vi "EnFlo_Seeder_Control.vi"(0 "Current Time (s)":dbl) -> ()   [LabVIEW 2021]
panel:
  in  "Minium Seeder power setting (Pmin)":dbl=27.0
  in  "Minimum Transducer Setting (Tmin)":dbl=6.0
  in  "Fluid Flowrate Factor":dbl=1.2 min=0.2 max=4.0 step=0.1 format="%.1g"
  in  "Sugar Strength":dbl=0.23
  out "Set All Outputs to Zero":bool
  in  "Performing hand clean":bool
  out "Run Transducer":bool
  out "Sugar Pump":bool
  out "Low Flow":bool
  out "High Flow":bool
  out "Time Since Last Flush (min)":dbl
  out "Running Flush time":dbl
  out "Transducer setting":dbl
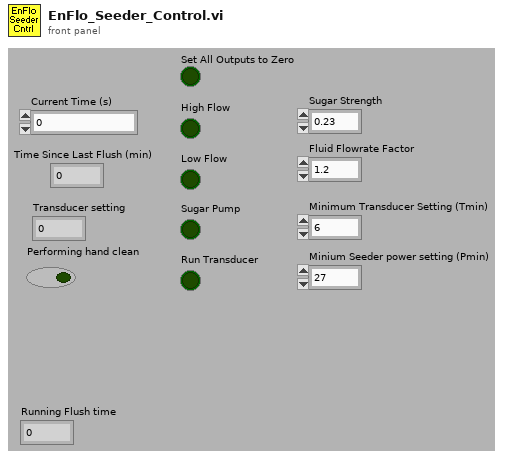
[diagram p1: front panel]
types:
  T1 = typedef "LVDateTimeRec.ctl" = cluster{"fractional second":dbl, "second":i32, "minute":i32, "hour":i32, "day of month":i32, "month":i32, "year":i32, "day of week":i32, "day of year":i32, "DST":i32}
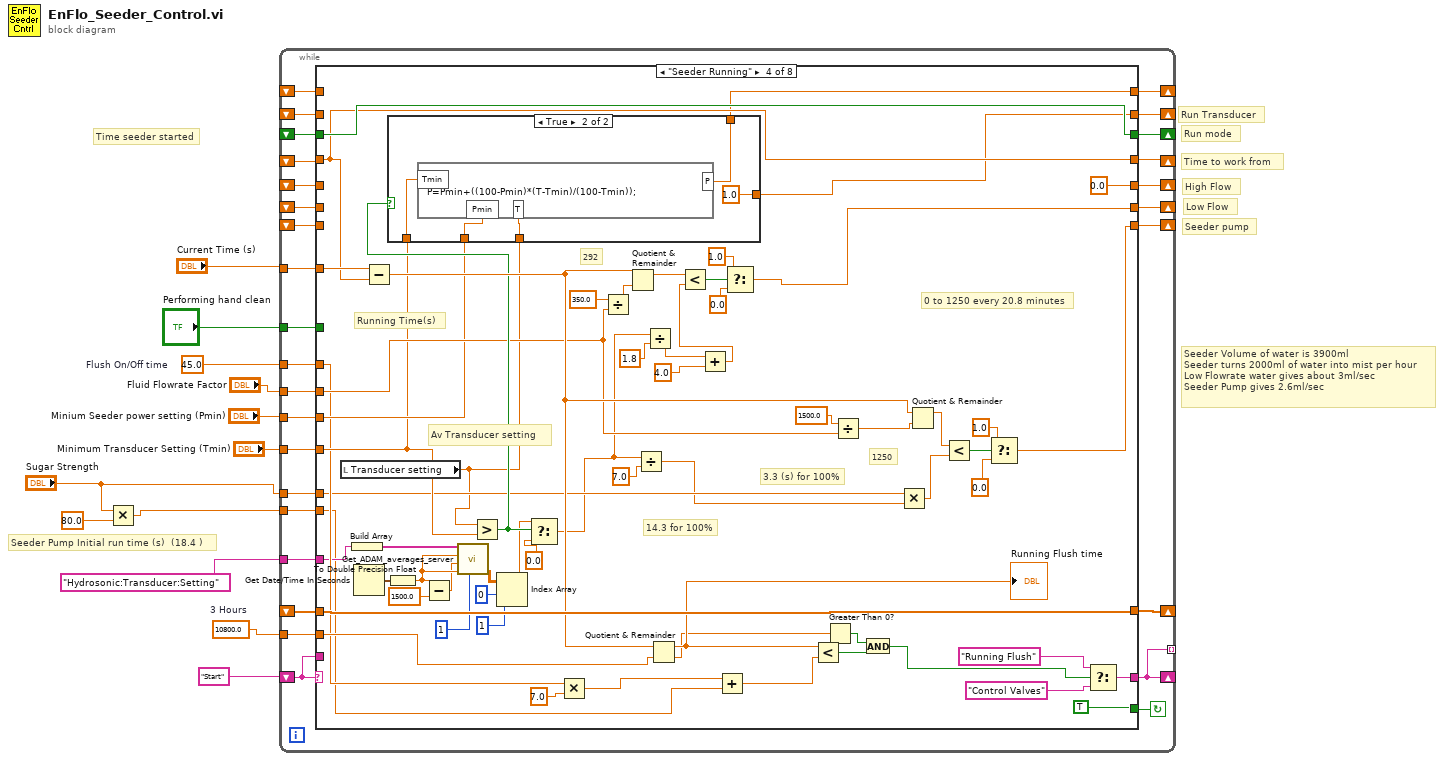
[diagram p0: block diagram]
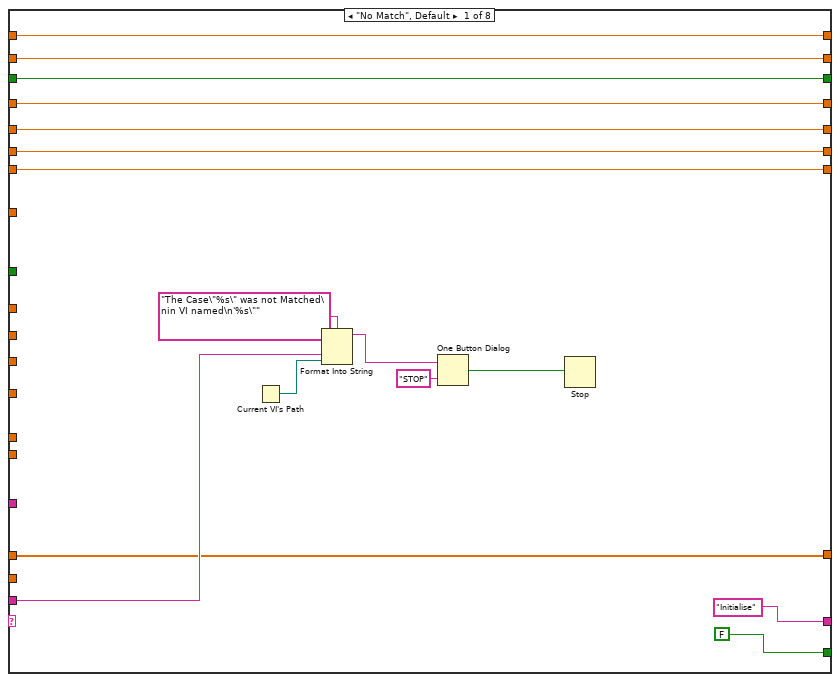
[diagram p2: hidden frame]
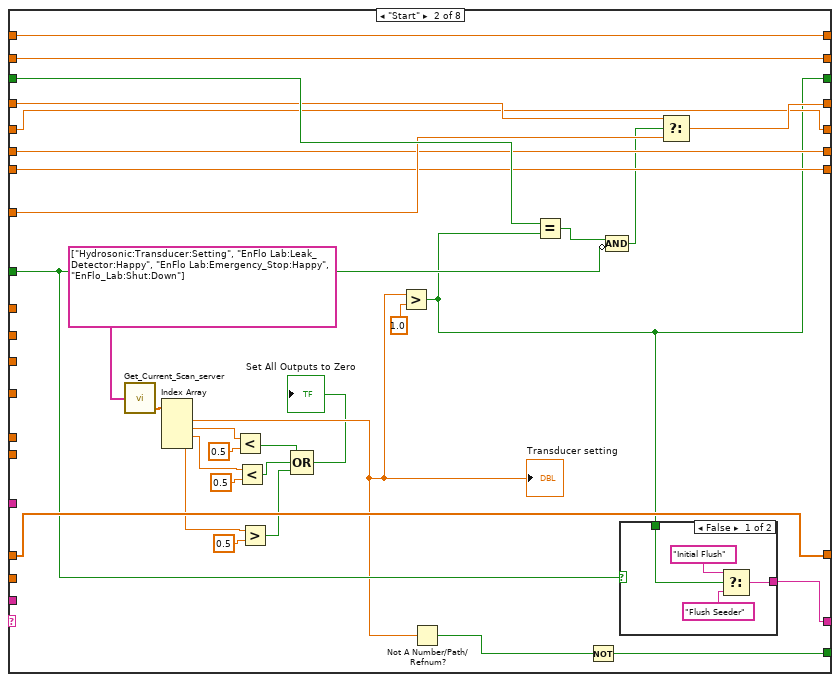
[diagram p3: hidden frame]
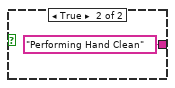
[diagram p4: hidden frame]
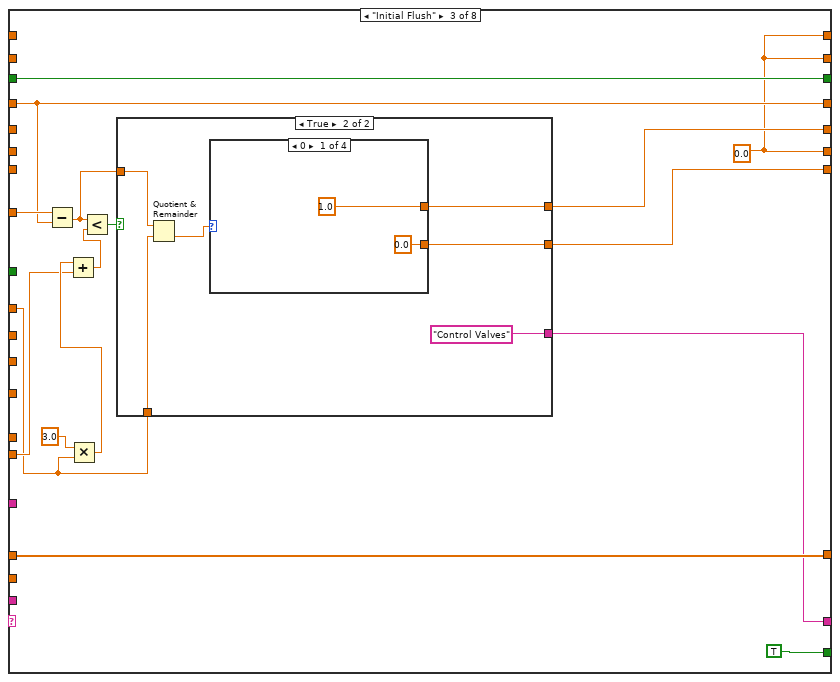
[diagram p5: hidden frame]
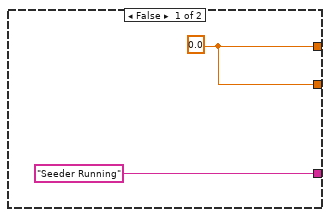
[diagram p6: hidden frame]
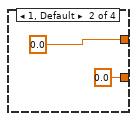
[diagram p7: hidden frame]
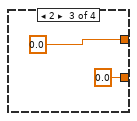
[diagram p8: hidden frame]
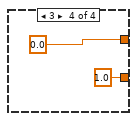
[diagram p9: hidden frame]
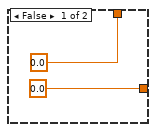
[diagram p10: hidden frame]
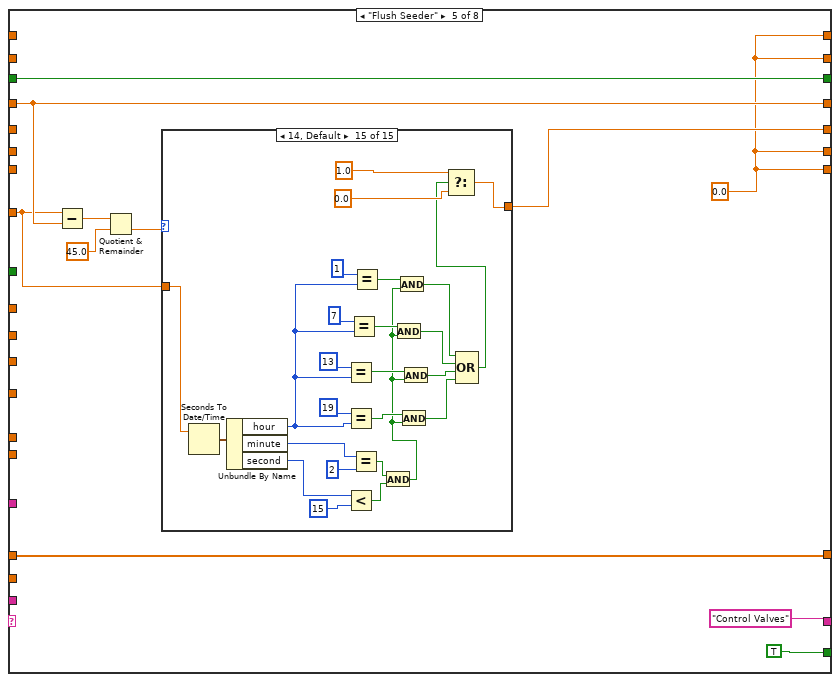
[diagram p11: hidden frame]
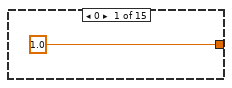
[diagram p12: hidden frame]
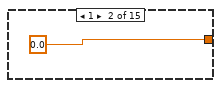
[diagram p13: hidden frame]
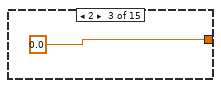
[diagram p14: hidden frame]
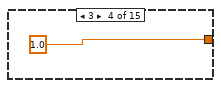
[diagram p15: hidden frame]
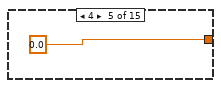
[diagram p16: hidden frame]
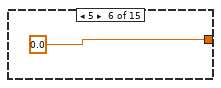
[diagram p17: hidden frame]
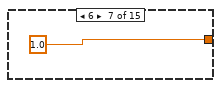
[diagram p18: hidden frame]
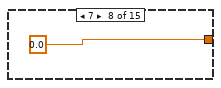
[diagram p19: hidden frame]
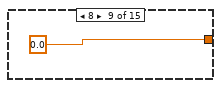
[diagram p20: hidden frame]
diagram:
  w5 = 45.0  # Flush On/Off time
  w10 = 10800.0  # 3 Hours
  # "Seeder Volume of water is 3900ml\nSeeder turns 2000ml of water into mist per hour\nLow Flowrate water gives about 3ml/sec\nSeeder Pump gives 2.6ml/sec"
  # "Seeder Pump Initial run time (s)  (18.4 )"
  # "Time seeder started"
  # "Run Transducer"
  # "Seeder pump"
  # "Low Flow"
  # "High Flow"
  # "Run mode"
  # "Time to work from"
  n1 = Multiply(x="Sugar Strength", y=80.0) -> (x*y=w1:dbl)
  n2 = while {
    shift-left: "Start" -> [w40]
    shift-right: [w24] -> _
    shift-right: [w39] -> _
    shift-left: _ -> [w36]
    shift-right: [w38] -> _
    shift-left: _ -> [w37]
    tunnel: "Current Time (s)" -> [w35]
    shift-right: [w33] -> _
    shift-left: _ -> [w34]
    shift-right: [w32] -> _
    shift-left: _ -> [w31]
    shift-right: [w29] -> _
    shift-left: _ -> [w30]
    shift-right: [w27] -> _
    shift-left: _ -> [w28]
    shift-right: [w26] -> _
    shift-left: _ -> [w25]
    tunnel: [w24] -> _ mode=indexing
    tunnel: w10 -> [w23]
    tunnel: "Performing hand clean" -> [w22]
    tunnel: "Sugar Strength" -> [w21]
    shift-right: [w20] -> _
    shift-left: _ -> [w19]
    tunnel: "Fluid Flowrate Factor" -> [w18]
    tunnel: "Minimum Transducer Setting (Tmin)" -> [w17]
    tunnel: "Minium Seeder power setting (Pmin)" -> [w16]
    tunnel: w5 -> [w15]
    tunnel: "Hydrosonic:Transducer:Setting" -> [w14]
    tunnel: w1 -> [w13]
    stop <- w41 continue-if-true
    n3 = case shown="\"Seeder Running\"" w40 {
      tunnel: [FALSE w86 TRUE TRUE TRUE TRUE TRUE FALSE] -> w41
      tunnel: ["Initialise" w81 w100 w168 "Control Valves" "Control Valves" "Control Valves" "End"] -> w24
      tunnel: w40 -> [w52 _ _ _ _ _ _ _]
      tunnel: [w47 w84 w103 w186 w203 w249 w263 w324] -> w39
      tunnel: [w49 w66 w108 w188 w204 w250 w264 w333] -> w38
      tunnel: w37 -> [w49 w85 w108 w188 w204 w250 w264 w333]
      tunnel: w36 -> [w47 w83 w103 w186 w203 w249 w263 w324]
      tunnel: w35 -> [_ w82 w104 w187 w196 _ _ w325]
      tunnel: w34 -> [w48 w80 _ _ _ _ _ w321]
      tunnel: [w48 w80 w107 0.0 w199 w247 w262 w321] -> w33
      tunnel: w31 -> [w46 w78 _ _ _ _ _ w319]
      tunnel: [w46 w78 w98 w176 w197 w247 w258 w319] -> w32
      tunnel: w30 -> [w45 w77 _ _ _ _ _ w317]
      tunnel: [w45 w77 w105 w171 w197 w247 w259 w317] -> w29
      tunnel: w28 -> [w44 w79 w106 w185 w198 w248 w261 w313]
      tunnel: [w44 w79 w106 w185 w198 w248 w261 w306] -> w27
      tunnel: w25 -> [w43 w76 _ _ _ _ _ w315]
      tunnel: [w43 w76 w98 w155 w197 w247 w258 w315] -> w26
      tunnel: w23 -> [_ _ _ w160 _ _ _ w309]
      tunnel: w22 -> [_ w73 _ _ _ _ _ _]
      tunnel: w21 -> [_ _ _ w134 _ _ _ _]
      tunnel: [w42 w69 w98 w154 w197 w247 w258 w301] -> w20
      tunnel: w19 -> [w42 w69 _ _ _ _ _ w301]
      tunnel: w18 -> [_ _ _ w150 _ _ _ _]
      tunnel: w17 -> [_ _ _ w147 _ _ _ _]
      tunnel: w16 -> [_ _ _ w148 _ _ _ _]
      tunnel: w15 -> [_ _ w94 w146 _ _ w257 _]
      tunnel: w14 -> [_ _ _ w143 _ _ _ _]
      tunnel: w13 -> [_ _ w95 w130 _ _ _ _]
      frame "No Match", Default {
        n4 = Current VI's Path() -> (path=w51:path)
        n5 = Format Into String(format string="The Case\"%s\" was not Matched\nin VI named\n'%s\"" ("Format String"), w52, w51) -> (resulting string=w55:string)  [unwired: 2 in, 1 out]
        n6 = One Button Dialog(message=w55, button name ("OK")="STOP") -> (true=w53:bool)
        n7 = Stop(stop? (T)=w53) -> ()
      }
      frame "Start" {
        n8 = call "Get_Current_Scan_server.vi"("Desired Channels"=string[] ["Hydrosonic:Transducer:Setting", "EnFlo Lab:Leak_Detector:Happy", "EnFlo Lab:Emergency_Stop:Happy", "EnFlo_Lab:Shut:Down"] ("appended array")) -> ("Numerical Values"=w88:dbl[])  [unwired: 2 out]
        n9 = Index Array(array=w88) -> (element #1=w68:dbl, element #2=w71:dbl, element #3=w64:dbl, element #4=w59:dbl)  [unwired: 4 in]
        "Transducer setting" <- w68
        n10 = Less?(x=w71, y=0.5) -> (x < y?=w62:bool)
        n11 = Less?(x=w64, y=0.5) -> (x < y?=w63:bool)
        n12 = Greater?(x=w59, y=0.5) -> (0:w58:bool)
        n13 = Compound Arithmetic op=OR(w62, w63, w58) -> (→"Set All Outputs to Zero":bool)
        n14 = Greater?(x=w68, y=1.0) -> (0:w66:bool)
        n15 = Not A Number/Path/Refnum?(number/path/refnum=w68) -> (NaN/Path/Refnum?=w87:bool)
        n16 = Equal?(x=w85, y=w66) -> (x = y?=w75:bool)
        n17 = Not(x=w87) -> (.not. x?=w86:bool)
        n18 = Compound Arithmetic op=AND(w75, invert w73) -> (w74:bool)
        n19 = case shown="False" w73 {
          tunnel: w66 -> [w92 _]
          tunnel: [w91 "Performing Hand Clean"] -> w81
          frame False {
            n20 = Select(t="Initial Flush", s=w92, f="Flush Seeder") -> (s? t:f=w91:string)
          }
          frame True {
          }
        }
        n21 = Select(t=w83, s=w74, f=w82) -> (s? t:f=w84:dbl)
      }
      frame "Initial Flush" {
        w98 = 0.0
        n22 = Subtract(x=w104, y=w103) -> (x-y=w101:dbl)
        n23 = Multiply(x=3.0, y=w94) -> (x*y=w96:dbl)
        n24 = Add(x=w96, y=w95) -> (x+y=w99:dbl)
        n25 = Less?(x=w101, y=w99) -> (x < y?=w102:bool)
        n26 = case shown="True" w102 {
          tunnel: [w111 w117] -> w107
          tunnel: [w111 w116] -> w105
          tunnel: w101 -> [_ w115]
          tunnel: ["Seeder Running" "Control Valves"] -> w100
          tunnel: w94 -> [_ w112]
          frame False {
            w111 = 0.0
          }
          frame True {
            n27 = Quotient & Remainder(x=w115, y=w112) -> (floor(x/y)=w114:dbl)  [unwired: 1 out]
            n28 = case shown="0" w114 {
              tunnel: [1.0 0.0 0.0 0.0] -> w117
              tunnel: [0.0 0.0 0.0 1.0] -> w116
              frame 0 {
              }
              frame 1, Default {
              }
              frame 2 {
              }
              frame 3 {
              }
            }
          }
        }
      }
      frame "Seeder Running" {
        # "3.3 (s) for 100%"
        # "14.3 for 100%"
        # "292"
        # "Av Transducer setting"
        # "0 to 1250 every 20.8 minutes"
        # "Running Time(s)"
        # "1250"
        n29 = local read "Transducer setting"() -> (w131:dbl)
        n30 = Build Array(w143) -> (w142:string[])
        n31 = Get Date/Time In Seconds() -> (seconds since 1Jan1904=w141:timestamp)
        n32 = Subtract(x=w187, y=w186) -> (x-y=w166:dbl)
        n33 = To Double Precision Float(number=w141) -> (double precision float=w140:dbl)
        n34 = Subtract(x=w140, y=1500.0) -> (x-y=w132:dbl)
        n35 = call "Get_ADAM_averages_server.vi"("No of averages"=1, "End time"=w140, "Start time"=w132, "Clients time"=w140, "ADAM Ch Names"=w142) -> ("DBL values"=w138:dbl[][])  [unwired: 1 in, 4 out]
        n36 = Greater?(x=w131, y=w147) -> (0:w156:bool)
        n37 = case shown="True" w156 {
          tunnel: [0.0 1.0] -> w155
          tunnel: [0.0 w192] -> w154
          tunnel: w148 -> [_ w194]
          tunnel: w147 -> [_ w193]
          tunnel: w131 -> [_ w191]
          frame False {
          }
          frame True {
            n38 = formula code="P=Pmin+((100-Pmin)*(T-Tmin)/(100-Tmin));"("Tmin"=w193, "T"=w191, "Pmin"=w194) -> ("P"=w192:dbl)
          }
        }
        n39 = Index Array(array=w138, index (row)=0, index (col)=1 ("disabled index (col)")) -> (element=w135:dbl)
        n40 = Select(t=w135, s=w156, f=0.0) -> (s? t:f=w128:dbl)
        n41 = Multiply(x=w146, y=7.0) -> (x*y=w144:dbl)
        n42 = Divide(x=350.0 ("y"), y=w150) -> (x/y=w152:dbl)
        n43 = Quotient & Remainder(x=w166, y=w152) -> (x-y*floor(x/y)=w184:dbl)  [unwired: 1 out]
        n44 = Divide(x=w128, y=7.0) -> (x/y=w129:dbl)
        n45 = Divide(x=w128, y=1.8) -> (x/y=w126:dbl)
        n46 = Quotient & Remainder(x=w166, y=w160) -> (x-y*floor(x/y)=w167:dbl, floor(x/y)=w164:dbl)
        "Running Flush time" <- w167
        n47 = Add(x=w126, y=4.0) -> (x+y=w179:dbl)
        n48 = Less?(x=w184, y=w179) -> (x < y?=w183:bool)
        n49 = Add(x=w144, y=w130) -> (x+y=w158:dbl)
        n50 = Select(t=1.0, s=w183, f=0.0) -> (s? t:f=w176:dbl)
        n51 = Less?(x=w167, y=w158) -> (x < y?=w162:bool)
        n52 = Greater Than 0?(x=w164) -> (x > 0?=w163:bool)
        n53 = Divide(x=1500.0 ("y"), y=w150) -> (x/y=w149:dbl)
        n54 = And(x=w163, y=w162) -> (x .and. y?=w161:bool)
        n55 = Multiply(x=w134, y=w129) -> (x*y=w159:dbl)
        n56 = Quotient & Remainder(x=w166, y=w149) -> (x-y*floor(x/y)=w172:dbl)  [unwired: 1 out]
        n57 = Less?(x=w172, y=w159) -> (x < y?=w173:bool)
        n58 = Select(t=1.0, s=w173, f=0.0) -> (s? t:f=w171:dbl)
        n59 = Select(t="Running Flush", s=w161, f="Control Valves") -> (s? t:f=w168:string)
      }
      frame "Flush Seeder" {
        w197 = 0.0
        n60 = Subtract(x=w196, y=w203) -> (x-y=w202:dbl)
        n61 = Quotient & Remainder(x=w202, y=45.0) -> (floor(x/y)=w200:dbl)  [unwired: 1 out]
        n62 = case shown="14, Default" w200 {
          tunnel: [1.0 0.0 0.0 1.0 0.0 0.0 1.0 0.0 0.0 1.0 0.0 0.0 1.0 0.0 w243] -> w199
          tunnel: w196 -> [_ _ _ _ _ _ _ _ _ _ _ _ _ _ w246]
          frame 0 {
          }
          frame 1 {
          }
          frame 2 {
          }
          frame 3 {
          }
          frame 4 {
          }
          frame 5 {
          }
          frame 6 {
          }
          frame 7 {
          }
          frame 8 {
          }
          frame 9 {
          }
          frame 10 {
          }
          frame 11 {
          }
          frame 12 {
          }
          frame 13 {
          }
          frame 14, Default {
            n63 = Seconds To Date/Time(time stamp (now)=w246) -> (date time rec=w242:T1)  [unwired: 1 in]
            n64 = Unbundle By Name(w242) -> ("hour"=w223:i32, "minute"=w240:i32, "second"=w238:i32)
            n65 = Equal?(x=13, y=w223) -> (x = y?=w230:bool)
            n66 = Equal?(x=19, y=w223) -> (x = y?=w232:bool)
            n67 = Less?(x=w238, y=15) -> (x < y?=w235:bool)
            n68 = Equal?(x=7, y=w223) -> (x = y?=w231:bool)
            n69 = Equal?(x=w240, y=2) -> (x = y?=w236:bool)
            n70 = Equal?(x=1, y=w223) -> (x = y?=w225:bool)
            n71 = And(x=w236, y=w235) -> (x .and. y?=w222:bool)
            n72 = And(x=w231, y=w222) -> (x .and. y?=w227:bool)
            n73 = And(x=w225, y=w222) -> (x .and. y?=w221:bool)
            n74 = And(x=w232, y=w222) -> (x .and. y?=w229:bool)
            n75 = And(x=w230, y=w222) -> (x .and. y?=w228:bool)
            n76 = Compound Arithmetic op=OR(w221, w227, w228, w229) -> (w226:bool)
            n77 = Select(t=1.0, s=w226, f=0.0) -> (s? t:f=w243:dbl)
          }
        }
      }
      frame "Performing Hand Clean" {
        w247 = 0.0
      }
      frame "Running Flush" {
        w258 = 0.0
        n78 = local read "Running Flush time"() -> (w260:dbl)
        n79 = Quotient & Remainder(x=w260, y=w257) -> (floor(x/y)=w256:dbl)  [unwired: 1 out]
        n80 = To Long Integer(number=w256) -> (32bit integer=w253:i32)
        n81 = feedback-in #1(w253) -> ()
        n82 = feedback #1() -> (w255:i32)  [unwired: 1 in]
        n83 = Not Equal?(x=w253, y=w255) -> (x != y?=w254:bool)
        n84 = case shown="7" w253 {
          tunnel: [1.0 0.0 1.0 0.0 1.0 0.0 0.0 0.0] -> w262
          tunnel: [0.0 0.0 0.0 0.0 0.0 0.0 0.0 w281] -> w259
          tunnel: w254 -> [_ _ _ _ _ _ _ w282]
          frame 0 {
          }
          frame 1 {
          }
          frame 2 {
          }
          frame 3 {
          }
          frame 4 {
          }
          frame 5, Default {
          }
          frame 6 {
          }
          frame 7 {
            n85 = local read "Transducer setting"() -> (w289:dbl)
            n86 = Less?(x=w289, y=5.5) -> (x < y?=w284:bool)
            n87 = case shown="True" w284 {
              tunnel: w289 -> [w297 _]
              tunnel: [w296 0.0 ("lower limit")] -> w283
              tunnel: [1.0 0.0] -> w281
              frame False {
                n88 = Add(x=w297, y=10.0) -> (x+y=w296:dbl)
              }
              frame True {
              }
            }
            n89 = In Range and Coerce(upper limit=100.0, x=w283, lower limit=0.0) -> (coerced(x)=w286:dbl)  [unwired: 1 out]
            n90 = case shown="True" w282 {
              tunnel: w286 -> [_ w291]
              frame False {
              }
              frame True {
                n91 = Build Array("Hydrosonic:Transducer:Setting") -> (w293:string[])
                n92 = Build Array(w291) -> (w292:dbl[])
                n93 = call "ASYNC_Adam_server.vi"("Values"=w292, "Channel Names"=w293) -> ()  [unwired: 1 in, 3 out]
              }
            }
          }
        }
      }
      frame "Control Valves" {
        n94 = Subtract(x=w325, y=w324) -> (x-y=w310:dbl)
        n95 = Quotient & Remainder(x=w310, y=w309) -> (x-y*floor(x/y)=w308:dbl)  [unwired: 1 out]
        n96 = Divide(x=w308, y=60.0) -> (x/y=→"Time Since Last Flush (min)":dbl)
        n97 = Build Array(w315, w321, w319, w317, w301) -> (w303:dbl[])
        n98 = Array Size(array=w313) -> (size(s)=w312:i32)
        n99 = local read "Set All Outputs to Zero"() -> (w307:bool)
        n100 = Equal To 0?(x=w312) -> (x = 0?=w311:bool)
        n101 = Array Size(array=w303) -> (size(s)=w305:i32)
        n102 = Initialize Array(0.0 ("element"), w305) -> (w302:dbl[])
        n103 = Select(t=w302, s=w307, f=w303) -> (s? t:f=w306:dbl[])
        n104 = case shown="True" w311 {
          tunnel: w306 -> [w338 w343]
          tunnel: string[] ["Hydrosonic:Seeder:Enable", "EnFlo_Tunnel:Seeder:High_Flow", "EnFlo_Tunnel:Seeder:Low_Flow", "EnFlo_Tunnel:Seeder_Pump:Enable", "EnFlo_Tunnel:Seeder:Power"] ("Desired Ch Names") -> [w337 w344]
          tunnel: [w336 w344] -> w329
          tunnel: [w335 w343] -> w328
          tunnel: w313 -> [w334 _]
          frame False {
            n105 = for {
              tunnel: w334 -> [w342] mode=indexing
              tunnel: w338 -> [w341] mode=indexing
              tunnel: [w341] -> w335 mode=indexing if=w339
              tunnel: w337 -> [w340] mode=indexing
              tunnel: [w340] -> w336 mode=indexing if=w339
              n106 = Not Equal?(x=w341, y=w342) -> (x != y?=w339:bool)
            }
          }
          frame True {
          }
        }
        n107 = Array Size(array=w328) -> (size(s)=w332:i32)
        n108 = Greater Than 0?(x=w332) -> (x > 0?=w331:bool)
        n109 = case shown="True" w331 {
          tunnel: w328 -> [_ w346]
          tunnel: w329 -> [_ w345]
          frame False {
          }
          frame True {
            n110 = call "ASYNC_Adam_server.vi"("Values"=w346, "Channel Names"=w345) -> ()  [unwired: 1 in, 3 out]
          }
        }
        n111 = Greater Than 0?(x=w321) -> (x > 0?=→"High Flow":bool)
        n112 = Greater Than 0?(x=w319) -> (x > 0?=→"Low Flow":bool)
        n113 = Greater Than 0?(x=w315) -> (x > 0?=→"Run Transducer":bool)
        n114 = Greater Than 0?(x=w317) -> (x > 0?=→"Sugar Pump":bool)
      }
    }
  }
